vi "Initialize DAQ RawDataQs.vi"(8 "error in (no error)":errorcluster, 11 "DAQ":refnum<class "DAQ.lvclass">) -> (0 "error out":errorcluster, 3 "DAQ":refnum<class "DAQ.lvclass">)   [LabVIEW 2022 SP3, in "DAQ.lvclass"]
doc: "Developed by Kevin Thompson\nkevin@thompsonengineering.net\n\nCopyright 2018-2020\nThompson Engineering, LLC"
uses:
  DAQ.lvclass
  DAQ.lvclass/DAQ.ctl
  Support/DataQueues/DataQueues.lvclass
  Support/DataQueues/DataTypes/DataQ SelectType--enum.ctl
  DataTypes/Dependency--cluster.ctl
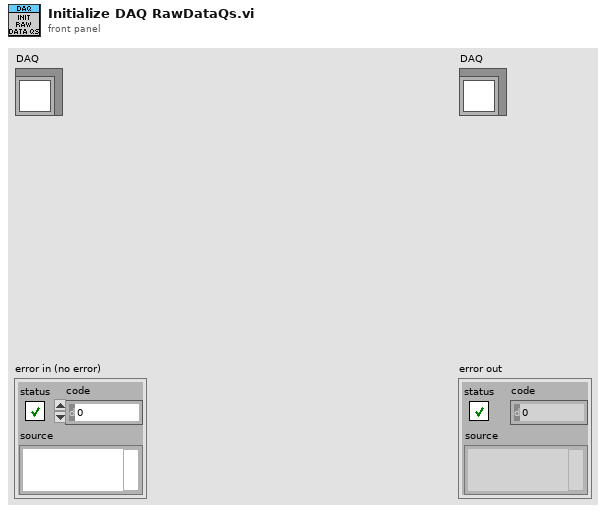
[diagram p1: front panel]
types:
  T1 = typedef "DAQ.lvclass/Dependency--cluster.ctl" = cluster{"DataQueues":refnum<class "DataQueues.lvclass">}
  T2 = typedef "DataQueues.lvclass/DataQ SelectType--enum.ctl" = enum16{"MainProcess", "LogEngine", "LocalDAQThread"}
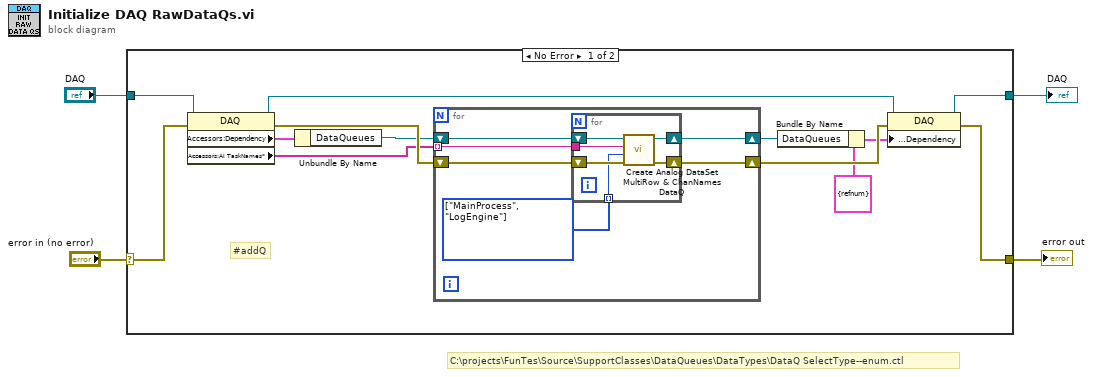
[diagram p0: block diagram]
diagram:
  # "C:\\projects\\FunTes\\Source\\SupportClasses\\DataQueues\\DataTypes\\DataQ SelectType--enum.ctl"
  n1 = case shown="No Error" "error in (no error)" {
    selector: "error in (no error)" -> [w16 w31]
    tunnel: "DAQ" -> [w13 w30]
    tunnel: [w10 w30] -> w3
    tunnel: [w17 w31] -> w2
    frame No Error {
      # "#addQ"
      n2 = property class="DAQ"(reference=w13, error in=w16) -> (reference out=w12:refnum<class "DAQ.lvclass">, error out=w15:errorcluster, "Accessors:Dependency"=w6:T1, "Accessors:AI TaskNames*"=w11:string[])
      n3 = Unbundle By Name(w6) -> ("DataQueues"=w5:refnum<class "DataQueues.lvclass">)
      n4 = for {
        shift-right: [w21] -> w8
        shift-left: w5 -> [w23]
        shift-right: [w22] -> w14
        shift-left: w15 -> [w20]
        tunnel: w11 -> [w19] mode=indexing
        w18 = T2[] [enum."MainProcess", enum."LogEngine"] items=["MainProcess", "LogEngine", "LocalDAQThread"]
        n5 = for {
          tunnel: w19 -> [w25]
          shift-right: [w29] -> w22
          shift-left: w20 -> [w27]
          shift-right: [w28] -> w21
          shift-left: w23 -> [w26]
          tunnel: w18 -> [w24] mode=indexing
          n6 = call "Create Analog DataSet MultiRow & ChanNames DataQ.vi"("error in (no error)"=w27, "Select"=w24, "TaskName"=w25, "DataQueues in"=w26) -> ("error out"=w29:errorcluster, "DataQueues out"=w28:refnum<class "DataQueues.lvclass">)  [unwired: 5 in, 1 out]
        }
      }
      n7 = Bundle By Name(cluster=T1 {"DataQueues"=refnum} ("Dependency"), "DataQueues"=w8) -> (w7:T1)
      n8 = property class="DAQ"(reference=w12, error in=w14, "Accessors:Dependency"=w7) -> (reference out=w10:refnum<class "DAQ.lvclass">, error out=w17:errorcluster)
    }
    frame Error {
    }
  }
  "error out" <- w2
  "DAQ" <- w3
